vi "Finish.vi"   [LabVIEW 2016]
doc: "This VI is called just before exiting. It is expected to close I/O refnum, save collected data, etc."
uses:
  <vilib>/Rock Robotics/WPI/Utilities/WPI_GetSetVariantRefNum.vi
types:
  T1 = typedef "WPI_SwitchDevRef.ctl" = cluster{"DevStatus":errorcluster, "DIO Channel":T2, "CntIndex":T3, "Normally Closed":bool}
  T2 = typedef "FPGA_DIOChannel.ctl" = enum8{"DIO 0", "DIO 1", "DIO 2", "DIO 3", "DIO 4", "DIO 5", "DIO 6", "DIO 7", "DIO 8", "DIO 9", "DIO MXP 0", "DIO MXP 1", "DIO MXP 2", "DIO MXP 3", "DIO MXP 4", "DIO MXP 5", "DIO MXP 6", "DIO MXP 7", "DIO MXP 8", "DIO MXP 9", "DIO MXP 10", "DIO MXP 11", "DIO MXP 12", "DIO MXP 13", "DIO MXP 14", "DIO MXP 15", "SPI Port CS1", "SPI Port CS2", "SPI Port CS3", "SPI Port MISO", "SPI Port MOSI", "Invalid"}
  T3 = typedef "FPGA_CounterCtrSystemIndex.ctl" = enum8{"Ctr 0", "Ctr 1", "Ctr 2", "Ctr 3", "Ctr 4", "Ctr 5", "Ctr 6", "Ctr 7", "Invalid"}
  T4 = typedef "WPI_SolenoidDevRef.ctl" = cluster{"DevStatus":errorcluster, "Pneumatics Control Module":u8, "Forward Solenoid Channel":T5, "Reverse Solenoid Channel":T5}
  T5 = typedef "WPI_SolenoidChannel.ctl" = enum8{"Solenoid 0", "Solenoid 1", "Solenoid 2", "Solenoid 3", "Solenoid 4", "Solenoid 5", "Solenoid 6", "Solenoid 7", "Invalid"}
  T6 = typedef "WPI_ServoDeviceRef.ctl" = cluster{"DeviceStatus":errorcluster, "PWM Channel":T7, "DeadBand":T8}
  T7 = typedef "FPGA_DIOPWMChannel.ctl" = enum8{"PWM 0", "PWM 1", "PWM 2", "PWM 3", "PWM 4", "PWM 5", "PWM 6", "PWM 7", "PWM 8", "PWM 9", "PWM MXP 0", "PWM MXP 1", "PWM MXP 2", "PWM MXP 3", "PWM MXP 4", "PWM MXP 5", "PWM MXP 6", "PWM MXP 7", "PWM MXP 8", "PWM MXP 9", "Invalid"}
  T8 = typedef "WPI_PWMDeadband.ctl" = cluster{"Name":string, "maxPositivePwm":i32, "minPositivePwm":i32, "centerPwm":i32, "maxNegativePwm":i32, "minNegativePwm":i32, "angularRange":u16}
  T9 = typedef "WPI_CounterDevRef.ctl" = cluster{"DevStatus":errorcluster, "CntIndex":T3}
  T10 = typedef "WPI_RelayDevRef.ctl" = cluster{"DevStatus":errorcluster, "Relay Channel":T11, "Relay Direction":T12}
  T11 = typedef "FPGA_DIORelayChannel.ctl" = enum8{"Relay 0", "Relay 1", "Relay 2", "Relay 3", "Invalid"}
  T12 = typedef "WPI_RelayDirection.ctl" = enum16{"Both directions", "Forward only", "Reverse only"}
  T13 = typedef "WPI_MotorControlDeviceRef.ctl" = cluster{"DeviceStatus":errorcluster, "Type":T14, "PWM":cluster{"PWM Channel":T7, "DeadBand":T8}, "CAN":cluster{"Device Number":u8, "SetOutput VI Ref":variant, "GetOutput VI Ref":variant, "Enable VI Ref":variant, "Disable VI Ref":variant, "Data":variant}, "Invert":bool}
  T14 = typedef "WPI_MotorControlType.ctl" = enum16{"PWM", "CAN"}
  T15 = typedef "WPI_I2CDevRef.ctl" = cluster{"DevStatus":errorcluster, "Device Address":u8, "Handle":i32, "I2C Bus":T16}
  T16 = typedef "i2c_bus.ctl" = enum16{"I2C On-Board", "I2C MXP", "Invalid"}
  T17 = typedef "WPI_JoystickDevRef.ctl" = cluster{"Device":T18}
  T18 = typedef "WPI_JoystickDeviceEnum.ctl" = enum16{"USB 0", "USB 1", "USB 2", "USB 3", "USB 4", "USB 5"}
  T19 = typedef "WPI_RobotDriveDevRef.ctl" = cluster{"DevStatus":errorcluster, "Motors[]":T13[], "Square Inputs":bool, "Max Output":dbl}
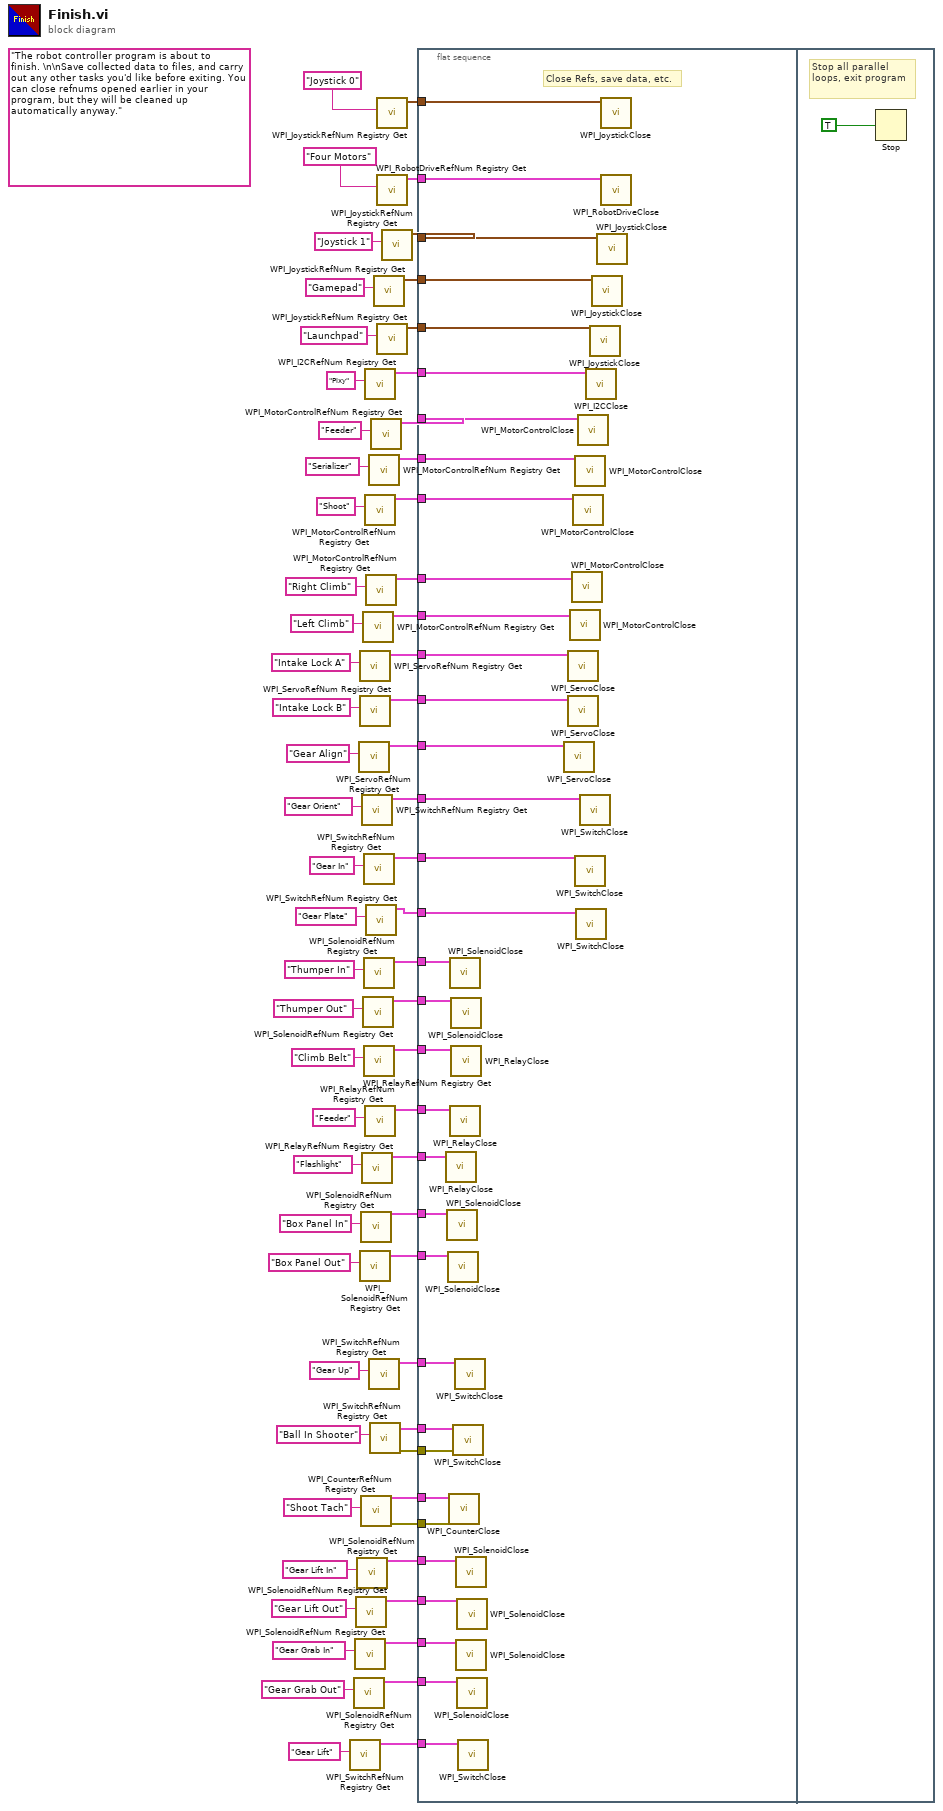
[diagram p0: block diagram]
diagram:
  (unwired) "The robot controller program is about to finish. \n\nSave collected data to files, and carry out any other tasks you'd like before exiting. You can close refnums opened earlier in your program, but they will be cleaned up automatically anyway."
  n1 = call <vilib>:"WPI_SwitchRefNum Registry Get.vi"("refnum name"="Gear Lift") -> ("SwitchDevRef"=w9:T1)  [unwired: 9 in, 1 out]
  n2 = call <vilib>:"WPI_SolenoidRefNum Registry Get.vi"("refnum name"="Gear Grab Out") -> ("SolenoidDevRef"=w11:T4)  [unwired: 9 in, 1 out]
  n3 = call <vilib>:"WPI_SolenoidRefNum Registry Get.vi"("refnum name"="Gear Grab In") -> ("SolenoidDevRef"=w12:T4)  [unwired: 9 in, 1 out]
  n4 = call <vilib>:"WPI_SolenoidRefNum Registry Get.vi"("refnum name"="Gear Lift Out") -> ("SolenoidDevRef"=w13:T4)  [unwired: 9 in, 1 out]
  n5 = call <vilib>:"WPI_SolenoidRefNum Registry Get.vi"("refnum name"="Gear Lift In") -> ("SolenoidDevRef"=w14:T4)  [unwired: 9 in, 1 out]
  n6 = call <vilib>:"WPI_ServoRefNum Registry Get.vi"("refnum name"="Gear Align") -> ("ServoDeviceRef"=w29:T6)  [unwired: 9 in, 1 out]
  n7 = call <vilib>:"WPI_ServoRefNum Registry Get.vi"("refnum name"="Intake Lock A") -> ("ServoDeviceRef"=w36:T6)  [unwired: 9 in, 1 out]
  n8 = call <vilib>:"WPI_ServoRefNum Registry Get.vi"("refnum name"="Intake Lock B") -> ("ServoDeviceRef"=w35:T6)  [unwired: 9 in, 1 out]
  n9 = call <vilib>:"WPI_SolenoidRefNum Registry Get.vi"("refnum name"="Box Panel Out") -> ("SolenoidDevRef"=w31:T4)  [unwired: 9 in, 1 out]
  n10 = call <vilib>:"WPI_SolenoidRefNum Registry Get.vi"("refnum name"="Box Panel In") -> ("SolenoidDevRef"=w34:T4)  [unwired: 9 in, 1 out]
  n11 = call <vilib>:"WPI_CounterRefNum Registry Get.vi"("refnum name"="Shoot Tach") -> ("error out"=w1:errorcluster, "CounterDevRef"=w2:T9)  [unwired: 9 in]
  n12 = call <vilib>:"WPI_SwitchRefNum Registry Get.vi"("refnum name"="Gear Orient") -> ("SwitchDevRef"=w50:T1)  [unwired: 9 in, 1 out]
  n13 = call <vilib>:"WPI_RelayRefNum Registry Get.vi"("refnum name"="Flashlight") -> ("RelayDevRef"=w39:T10)  [unwired: 9 in, 1 out]
  n14 = call <vilib>:"WPI_MotorControlRefNum Registry Get.vi"("refnum name"="Left Climb") -> ("MotorControlDevRef"=w23:T13)  [unwired: 9 in, 1 out]
  n15 = call <vilib>:"WPI_SolenoidRefNum Registry Get.vi"("refnum name"="Thumper Out") -> ("SolenoidDevRef"=w19:T4)  [unwired: 9 in, 1 out]
  n16 = call <vilib>:"WPI_SwitchRefNum Registry Get.vi"("refnum name"="Gear In") -> ("SwitchDevRef"=w49:T1)  [unwired: 9 in, 1 out]
  n17 = call <vilib>:"WPI_SolenoidRefNum Registry Get.vi"("refnum name"="Thumper In") -> ("SolenoidDevRef"=w20:T4)  [unwired: 9 in, 1 out]
  n18 = call <vilib>:"WPI_RelayRefNum Registry Get.vi"("refnum name"="Climb Belt") -> ("RelayDevRef"=w44:T10)  [unwired: 9 in, 1 out]
  n19 = call <vilib>:"WPI_I2CRefNum Registry Get.vi"("refnum name"="Pixy") -> ("I2CDevRef"=w52:T15)  [unwired: 9 in, 1 out]
  n20 = call <vilib>:"WPI_MotorControlRefNum Registry Get.vi"("refnum name"="Shoot") -> ("MotorControlDevRef"=w28:T13)  [unwired: 9 in, 1 out]
  n21 = call <vilib>:"WPI_RelayRefNum Registry Get.vi"("refnum name"="Feeder") -> ("RelayDevRef"=w41:T10)  [unwired: 9 in, 1 out]
  n22 = call <vilib>:"WPI_MotorControlRefNum Registry Get.vi"("refnum name"="Right Climb") -> ("MotorControlDevRef"=w27:T13)  [unwired: 9 in, 1 out]
  n23 = call <vilib>:"WPI_SwitchRefNum Registry Get.vi"("refnum name"="Gear Plate") -> ("SwitchDevRef"=w48:T1)  [unwired: 9 in, 1 out]
  n24 = call <vilib>:"WPI_MotorControlRefNum Registry Get.vi"("refnum name"="Serializer") -> ("MotorControlDevRef"=w56:T13)  [unwired: 9 in, 1 out]
  n25 = call <vilib>:"WPI_SwitchRefNum Registry Get.vi"("refnum name"="Gear Up") -> ("SwitchDevRef"=w7:T1)  [unwired: 9 in, 1 out]
  n26 = call <vilib>:"WPI_SwitchRefNum Registry Get.vi"("refnum name"="Ball In Shooter") -> ("error out"=w4:errorcluster, "SwitchDevRef"=w5:T1)  [unwired: 9 in]
  n27 = call <vilib>:"WPI_MotorControlRefNum Registry Get.vi"("refnum name"="Feeder") -> ("MotorControlDevRef"=w55:T13)  [unwired: 9 in, 1 out]
  n28 = call <vilib>:"WPI_JoystickRefNum Registry Get.vi"("refnum name"="Gamepad") -> ("JoystickDevRef"=w61:T17)  [unwired: 9 in, 1 out]
  n29 = call <vilib>:"WPI_JoystickRefNum Registry Get.vi"("refnum name"="Joystick 0") -> ("JoystickDevRef"=w63:T17)  [unwired: 1 in, 9 out]
  n30 = call <vilib>:"WPI_RobotDriveRefNum Registry Get.vi"("refnum name"="Four Motors") -> ("RobotDriveDevRef"=w64:T19)  [unwired: 1 in, 9 out]
  n31 = call <vilib>:"WPI_JoystickRefNum Registry Get.vi"("refnum name"="Launchpad") -> ("JoystickDevRef"=w62:T17)  [unwired: 9 in, 1 out]
  n32 = call <vilib>:"WPI_JoystickRefNum Registry Get.vi"("refnum name"="Joystick 1") -> ("JoystickDevRef"=w60:T17)  [unwired: 9 in, 1 out]
  n33 = flat-sequence {
    tunnel: w64 -> [w100]
    tunnel: w63 -> [w99]
    tunnel: w62 -> [w98]
    tunnel: w61 -> [w97]
    tunnel: w60 -> [w96]
    tunnel: w56 -> [w95]
    tunnel: w55 -> [w94]
    tunnel: w52 -> [w93]
    tunnel: w50 -> [w92]
    tunnel: w49 -> [w91]
    tunnel: w48 -> [w90]
    tunnel: w44 -> [w89]
    tunnel: w41 -> [w88]
    tunnel: w39 -> [w87]
    tunnel: w36 -> [w86]
    tunnel: w35 -> [w85]
    tunnel: w34 -> [w84]
    tunnel: w31 -> [w83]
    tunnel: w29 -> [w82]
    tunnel: w28 -> [w81]
    tunnel: w27 -> [w80]
    tunnel: w23 -> [w79]
    tunnel: w20 -> [w78]
    tunnel: w19 -> [w77]
    tunnel: w14 -> [w76]
    tunnel: w13 -> [w75]
    tunnel: w12 -> [w74]
    tunnel: w11 -> [w73]
    tunnel: w9 -> [w72]
    tunnel: w7 -> [w71]
    tunnel: w5 -> [w70]
    tunnel: w4 -> [w69]
    tunnel: w2 -> [w68]
    tunnel: w1 -> [w67]
    frame #0 {
      # "Close Refs, save data, etc."
      n34 = call <vilib>:"WPI_RelayClose.vi"("RelayDevRef"=w87) -> ()  [unwired: 10 in, 1 out]
      n35 = call <vilib>:"WPI_SolenoidClose.vi"("SolenoidDevRef"=w84) -> ()  [unwired: 10 in, 1 out]
      n36 = call <vilib>:"WPI_SolenoidClose.vi"("SolenoidDevRef"=w83) -> ()  [unwired: 10 in, 1 out]
      n37 = call <vilib>:"WPI_CounterClose.vi"("error in (no error)"=w67, "CounterDevRef"=w68) -> ()  [unwired: 9 in, 1 out]
      n38 = call <vilib>:"WPI_SolenoidClose.vi"("SolenoidDevRef"=w78) -> ()  [unwired: 10 in, 1 out]
      n39 = call <vilib>:"WPI_RelayClose.vi"("RelayDevRef"=w88) -> ()  [unwired: 10 in, 1 out]
      n40 = call <vilib>:"WPI_SolenoidClose.vi"("SolenoidDevRef"=w77) -> ()  [unwired: 10 in, 1 out]
      n41 = call <vilib>:"WPI_RelayClose.vi"("RelayDevRef"=w89) -> ()  [unwired: 10 in, 1 out]
      n42 = call <vilib>:"WPI_SwitchClose.vi"("error in (no error)"=w69, "SwitchDevRef"=w70) -> ()  [unwired: 9 in, 1 out]
      n43 = call <vilib>:"WPI_SwitchClose.vi"("SwitchDevRef"=w71) -> ()  [unwired: 10 in, 1 out]
      n44 = call <vilib>:"WPI_SolenoidClose.vi"("SolenoidDevRef"=w76) -> ()  [unwired: 10 in, 1 out]
      n45 = call <vilib>:"WPI_SolenoidClose.vi"("SolenoidDevRef"=w74) -> ()  [unwired: 10 in, 1 out]
      n46 = call <vilib>:"WPI_SolenoidClose.vi"("SolenoidDevRef"=w75) -> ()  [unwired: 10 in, 1 out]
      n47 = call <vilib>:"WPI_SolenoidClose.vi"("SolenoidDevRef"=w73) -> ()  [unwired: 10 in, 1 out]
      n48 = call <vilib>:"WPI_SwitchClose.vi"("SwitchDevRef"=w72) -> ()  [unwired: 10 in, 1 out]
      n49 = call <vilib>:"WPI_ServoClose.vi"("ServoDeviceRef"=w82) -> ()  [unwired: 10 in, 1 out]
      n50 = call <vilib>:"WPI_ServoClose.vi"("ServoDeviceRef"=w86) -> ()  [unwired: 10 in, 1 out]
      n51 = call <vilib>:"WPI_ServoClose.vi"("ServoDeviceRef"=w85) -> ()  [unwired: 10 in, 1 out]
      n52 = call <vilib>:"WPI_MotorControlClose.vi"("MotorControlDevRef"=w79) -> ()  [unwired: 10 in, 1 out]
      n53 = call <vilib>:"WPI_MotorControlClose.vi"("MotorControlDevRef"=w80) -> ()  [unwired: 10 in, 1 out]
      n54 = call <vilib>:"WPI_MotorControlClose.vi"("MotorControlDevRef"=w81) -> ()  [unwired: 10 in, 1 out]
      n55 = call <vilib>:"WPI_MotorControlClose.vi"("MotorControlDevRef"=w95) -> ()  [unwired: 10 in, 1 out]
      n56 = call <vilib>:"WPI_SwitchClose.vi"("SwitchDevRef"=w91) -> ()  [unwired: 10 in, 1 out]
      n57 = call <vilib>:"WPI_SwitchClose.vi"("SwitchDevRef"=w90) -> ()  [unwired: 10 in, 1 out]
      n58 = call <vilib>:"WPI_MotorControlClose.vi"("MotorControlDevRef"=w94) -> ()  [unwired: 10 in, 1 out]
      n59 = call <vilib>:"WPI_SwitchClose.vi"("SwitchDevRef"=w92) -> ()  [unwired: 10 in, 1 out]
      n60 = call <vilib>:"WPI_I2CClose.vi"("I2CDevRef"=w93) -> ()  [unwired: 10 in, 1 out]
      n61 = call <vilib>:"WPI_JoystickClose.vi"("JoystickDevRef"=w98) -> ()  [unwired: 11 in]
      n62 = call <vilib>:"WPI_JoystickClose.vi"("JoystickDevRef"=w97) -> ()  [unwired: 11 in]
      n63 = call <vilib>:"WPI_JoystickClose.vi"("JoystickDevRef"=w96) -> ()  [unwired: 11 in]
      n64 = call <vilib>:"WPI_JoystickClose.vi"("JoystickDevRef"=w99) -> ()  [unwired: 11 out]
      n65 = call <vilib>:"WPI_RobotDriveClose.vi"("RobotDriveDevRef"=w100) -> ()  [unwired: 1 in, 10 out]
    }
    frame #1 {
      # "Stop all parallel\nloops, exit program"
      n66 = Stop(stop? (T)=TRUE ("Quit")) -> ()
    }
  }
